vi "TDT-Close.vi"(0 "Data":T1={"TTankX"=refnum, "TDevAccX"=refnum, "LastTime"=0.0, "error"={"status"=FALSE, "code"=0, "source"=""}, "Block Name"="", "Circuit Tag"="", "Tank Name"="", "NumTicks"=0, "LastTick"=0.0, "Idle?"=FALSE, "Wait (ms)"=1000, "LastArtf"=0.0, "LastTosc"=0.0}, 11 "error in (no error)":errorcluster) -> (4 "Data out":T1={"TTankX"=refnum, "TDevAccX"=refnum, "LastTime"=0.0, "error"={"status"=FALSE, "code"=0, "source"=""}, "Block Name"="", "Circuit Tag"="", "Tank Name"="", "NumTicks"=0, "LastTick"=0.0, "Idle?"=FALSE, "Wait (ms)"=1000, "LastArtf"=0.0, "LastTosc"=0.0}, 15 "error out":errorcluster)   [LabVIEW 2015]
uses:
  TDT Interface Data.ctl
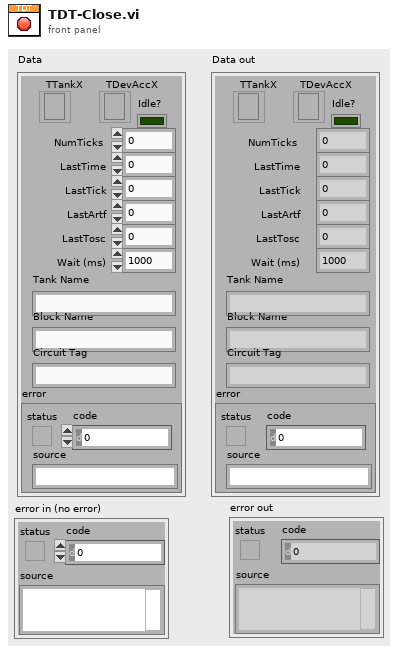
[diagram p1: front panel]
types:
  T1 = typedef "TDT Interface Data.ctl" = cluster{"TTankX":refnum<k7>, "TDevAccX":refnum<k7>, "LastTime":dbl, "error":errorcluster, "Block Name":string, "Circuit Tag":string, "Tank Name":string, "NumTicks":i32, "LastTick":dbl, "Idle?":bool, "Wait (ms)":u32, "LastArtf":dbl, "LastTosc":dbl}
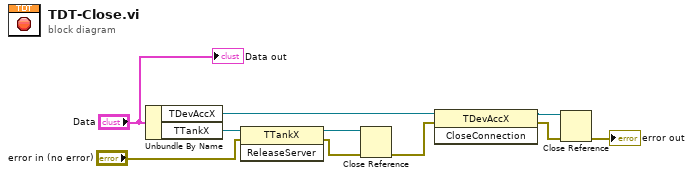
[diagram p0: block diagram]
diagram:
  n1 = Unbundle By Name("Data") -> ("TDevAccX"=w6:refnum<k7>, "TTankX"=w10:refnum<k7>)
  n2 = invoke class="TTankX" method="ReleaseServer"(reference=w10, error in="error in (no error)") -> (reference out=w9:refnum<k7>, error out=w8:errorcluster)  [unwired: 1 in, 1 out]
  n3 = Close Reference(reference=w9, error in (no error)=w8) -> (error out=w5:errorcluster)
  n4 = invoke class="TDevAccX" method="CloseConnection"(reference=w6, error in=w5) -> (reference out=w4:refnum<k7>, error out=w3:errorcluster)  [unwired: 1 in, 1 out]
  n5 = Close Reference(reference=w4, error in (no error)=w3) -> (error out=→"error out":errorcluster)
  "Data out" <- "Data"
